vi "WPI_SimpleGyro_RefNum Registry Get.vi"(8 "error in (no error)":errorcluster, 11 "refnum name":string="SimpleGyroRefNum") -> (0 "error out":errorcluster, 3 "SimpleGyroDevRef":T1)   [LabVIEW 2014, in "SimpleGyro.lvlib"]
doc: "Use this to get the reference you specify. You first must set the reference using RefNum Registry Set.vi."
uses:
  SimpleGyro.lvlib
  WPI_SimpleGyroDevRef.ctl
  <vilib>/Rock Robotics/SystemInterfaces/Typedef/FPGA_TypedefDigitalModule.ctl
  <vilib>/Rock Robotics/SystemInterfaces/spilib/spi_bus.ctl
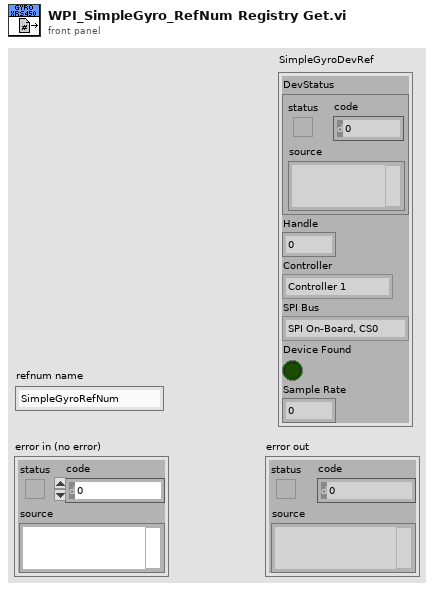
[diagram p1: front panel]
types:
  T1 = typedef "SimpleGyro.lvlib/WPI_SimpleGyroDevRef.ctl" = cluster{"DevStatus":errorcluster, "Handle":i32, "Controller":T2, "SPI Bus":T3, "Device Found":bool, "Sample Rate":dbl}
  T2 = typedef "FPGA_TypedefDigitalModule.ctl" = enum16{"Controller 1"}
  T3 = typedef "spi_bus.ctl" = enum16{"SPI On-Board, CS0", "SPI On-Board, CS1", "SPI On-Board, CS2", "SPI On-Board, CS3", "SPI MXP", "Invalid"}
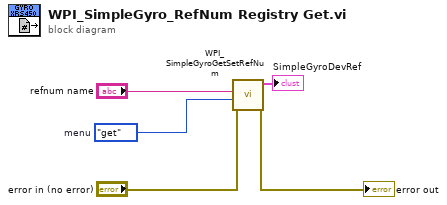
[diagram p0: block diagram]
diagram:
  w3 = enum16{"set", "get", "delete"}."get"  # menu
  n1 = call "WPI_SimpleGyroGetSetRefNum.vi"("error in (no error)"="error in (no error)", "menu"=w3, "refnum name"="refnum name") -> ("error out"=→"error out":errorcluster, "SimpleGyroDevRef"=→"SimpleGyroDevRef":T1)  [unwired: 7 in]
